vi "SENS_MULT_ALLP.vi"(0 "VISA IN":refnum<visa-resource-name>, 1 "ID":i32, 2 "Port Selections":string, 5 "error in":errorcluster, 7 "Channel":i32) -> (14 "VISA Out":refnum<visa-resource-name>, 19 "error out":errorcluster)   [LabVIEW 2018, in "PNA-X.lvlib"]
doc: "SENSe<cnum>:MULTiplexer<id>:ALLPorts <string> \n(Read-Write) Sets or gets the port selections for all available ports on the specified channel. \nParameters \n<cnum> Any existing channel number. If unspecified, value is set to 1. \n<id> Id of the external test set. If unspecified, Id is assumed to be 1. Must be \npreviously set by the SENSe:MULT:TYPE command. \n<string> Comma-separated list of port selections, one for each port. Each port selection \nmust correspond to one of the values returned by SENS:MULT:PORT:CAT?. \nDo NOT include + and - . \nExamples ' for channel 5 and test set 1, set port 1 to T1, \n' port 2 to A, port 3 to R2+, port 4 to R3-. \nSENS5:MULT1:ALLP \"T1,A,R2,R3 \" \nQuery Syntax SENSe<cnum>:MULTiplexer<id>:ALLPorts? \nReturn Type STRING \nDefault Not Applicable \nSENSe:MULTiplexer:CATalog? \n(Read-Only) Returns a comma-separated list of the external test sets models that are currently \nsupported. Choose one of these items to send SENS:MULT1:TYPE. \nExamples SENS:MULT:CAT? \nReturn Type String \nDefault Not Applicable \n1780\n\nSENSe:MULTiplexer<id>:COUNt? \n(Read-Only) Returns the total number of ports of the specified test set. \nReturns 0 if no test set is connected (GPIB test sets only). \nParameters \n<id> Id of the external test set. If unspecified, Id is assumed to be 1. Must be \npreviously set by the SENSe:MULT:TYPE command. \nExamples SENS:MULT1:COUN? \nsense:multiplexer2:count? \nReturn Type Numeric \nDefault Not Applicable \nSENSe:MULTiplexer<id>:DISPlay[:STATe] <bool> \n(Read-Write) Turns ON and OFF the display of the test set control status bar. This status bar indicates \nthe test set that is being controlled and the current port mappings. This setting is turned ON \nautomatically when the test set is enabled. \nParameters \n<id> Id of the external test set. If unspecified, Id is assumed to be 1. Must be \npreviously set by the SENSe:MULT:TYPE command. \n<bool> ON(1) Turns ON the display. \nOFF (0) Turns OFF the display. \nExamples SENS:MULT1:DISP 1 \nsense:multiplexer2:display:state on \nQuery Syntax SENSe:MULTiplexer<id>:DISPlay[:STATe]? \nReturn Type Boolean \nDefault OFF (0) \nSENSe:MULTiplexer<id>:INCount? \n1781\n\n(Read-Only) Returns the number of input ports for the specified test set. \nFor test sets such as the E5091A that do NOT use jumper cables to route the stimulus and response signals, \nthis command returns the number of test set ports that can be connected to the PNA. \nFor test sets that DO use jumper cables to route the stimulus and response signals, such as the N44xx, the \nreturn value is not valid. \nParameters \n<id> Id of the external test set. If unspecified, Id is assumed to be 1. Must be \npreviously set by the SENSe:MULT:TYPE command. \nExamples SENS3:MULT1:INC? ' returns the number of input ports for test \nset 1 on channel 3 \nReturn Type Numeric \nDefault Not Applicable"
uses:
  PNA-X.lvlib
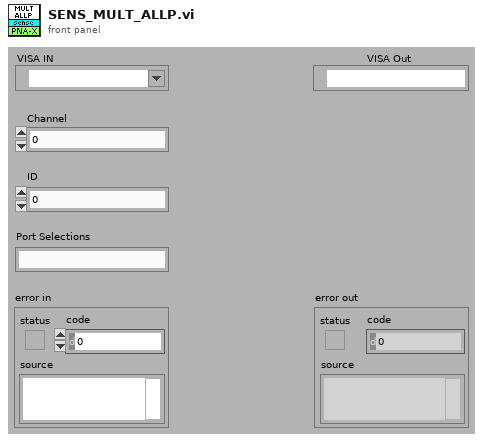
[diagram p1: front panel]
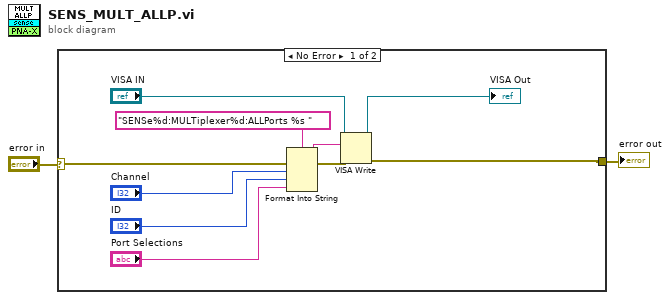
[diagram p0: block diagram]
diagram:
  n1 = case shown="No Error" "error in" {
    selector: "error in" -> [w12 w13]
    tunnel: [w7 w13] -> w1
    frame No Error {
      n2 = Format Into String(format string="SENSe%d:MULTiplexer%d:ALLPorts %s " ("Cmdline"), error in=w12, "Channel", "ID", "Port Selections") -> (resulting string=w10:string, error out=w11:errorcluster)  [unwired: 1 in]
      n3 = VISA Write(VISA resource name="VISA IN", write buffer=w10, error in (no error)=w11) -> (VISA resource name out=→"VISA Out":refnum<visa-resource-name>, error out=w7:errorcluster)  [unwired: 1 out]
    }
    frame Error {
    }
  }
  "error out" <- w1
